vi "2283_LEDControllers.vi"() -> ()   [LabVIEW 2014]
panel:
  in  "LED controllers":T1
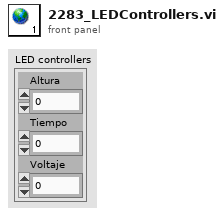
[diagram p1: front panel]
types:
  T1 = cluster{"Altura":dbl, "Tiempo":dbl, "Voltaje":dbl}
diagram:
